vi "Read Multi Eval Meas ES Flatness Results.vi"(8 "error in (no error)":errorcluster, 9 "Result Type (Current)":i32(ring) items=["Current", "Average", "Extreme", "Standard Deviation"], 10 "Instance (1)":T2=1, 11 "VISA resource name":refnum<visa-resource-name>) -> (0 "error out":errorcluster, 1 "Flatness Results":T1 {"Max R2" format="%^.3e"; "Min R2" format="%^.3e"; "Max R1" format="%^.3e"; "Min R1" format="%^.3e"; "Max R2 Min R1" format="%^.3e"; "Max R1 Min R2" format="%^.3e"; "Ripple 2" format="%^.3e"; "Ripple 1" format="%^.3e"}, 2 "Reliability":i32, 3 "VISA resource name out":refnum<visa-resource-name>, 5 "Out Of Tolerance":i32)   [LabVIEW 2020, in "Rohde&Schwarz CMWXP NR FR1 Measurement.lvlib"]
doc: "Return current, average, extreme and standard deviation single value results of the equalizer spectrum flatness measurement.\n\nAttributes:\nRSCMWXPNRFR1M_ATTR_READ_MULTI_EVAL_MEAS_ES_FLATNESS_CURRENT_RESULTS\nRSCMWXPNRFR1M_ATTR_READ_MULTI_EVAL_MEAS_ES_FLATNESS_AVERAGE_RESULTS\nRSCMWXPNRFR1M_ATTR_READ_MULTI_EVAL_MEAS_ES_FLATNESS_EXTREME_RESULTS\nRSCMWXPNRFR1M_ATTR_READ_MULTI_EVAL_MEAS_ES_FLATNESS_STANDARD_DEVIATION_RESULTS\n\nRemote-control commands:\nREAD:NRSub:MEAS<i>:MEValuation:ESFLatness:CURRent?\nREAD:NRSub:MEAS<i>:MEValuation:ESFLatness:AVERage?\nREAD:NRSub:MEAS<i>:MEValuation:ESFLatness:EXTReme?\nREAD:NRSub:MEAS<i>:MEValuation:ESFLatness:SDEViation?"
uses:
  <instrlib>/Rohde&Schwarz CMWXP NR FR1 Measurement/Rohde&Schwarz CMWXP NR FR1 Measurement.lvlib
  <instrlib>/Rohde&Schwarz CMWXP NR FR1 Measurement/Private/_Instance.ctl
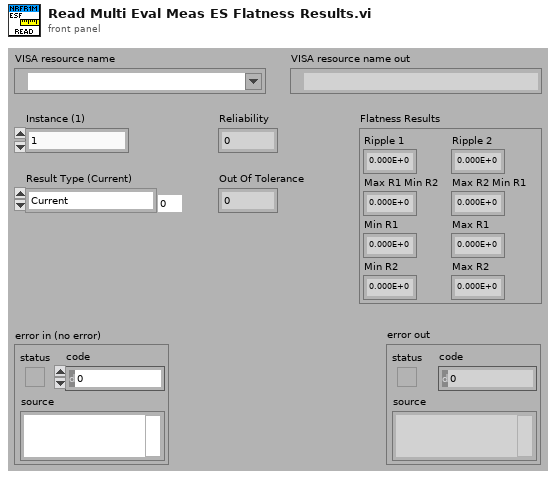
[diagram p1: front panel]
types:
  T1 = cluster{"Ripple 1":dbl, "Ripple 2":dbl, "Max R1 Min R2":dbl, "Max R2 Min R1":dbl, "Min R1":dbl, "Max R1":dbl, "Min R2":dbl, "Max R2":dbl}
  T2 = typedef "Rohde&Schwarz CMWXP NR FR1 Measurement.lvlib/_Instance.ctl" = i32
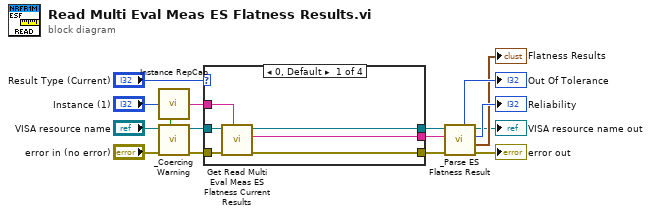
[diagram p0: block diagram]
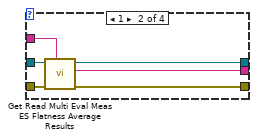
[diagram p2: hidden frame]
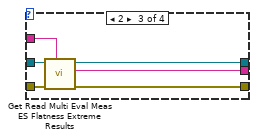
[diagram p3: hidden frame]
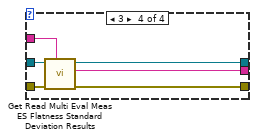
[diagram p4: hidden frame]
diagram:
  n1 = call <instrlib>:"Instance RepCap.vi"("Instance In"="Instance (1)") -> ("In Range?"=w14:bool, "RepCap Identifier Out"=w12:string)  [unwired: 1 in]
  n2 = call <instrlib>:"_Coercing Warning.vi"("In Range?"=w14, "error in (no error)"="error in (no error)", "VISA resource name"="VISA resource name") -> ("error out"=w10:errorcluster, "VISA resource name out"=w11:refnum<visa-resource-name>)  [unwired: 7 in]
  n3 = case shown="0, Default" "Result Type (Current)" {
    tunnel: w12 -> [w22 w28 w34 w40]
    tunnel: w11 -> [w21 w27 w33 w39]
    tunnel: w10 -> [w20 w26 w32 w38]
    tunnel: [w19 w25 w31 w37] -> w6
    tunnel: [w18 w24 w30 w36] -> w7
    tunnel: [w17 w23 w29 w35] -> w8
    frame 0, Default {
      n4 = call "Get Read Multi Eval Meas ES Flatness Current Results"("Repeated Capabilities"=w22, "error in (no error)"=w20, "instrument handle"=w21) -> ("error out"=w17:errorcluster, "Read Multi Eval Meas ES Flatness Current Results"=w18:string, "instrument handle out"=w19:refnum<visa-resource-name>)  [unwired: 6 in]
    }
    frame 1 {
      n5 = call "Get Read Multi Eval Meas ES Flatness Average Results"("Repeated Capabilities"=w28, "error in (no error)"=w26, "instrument handle"=w27) -> ("error out"=w23:errorcluster, "Read Multi Eval Meas ES Flatness Average Results"=w24:string, "instrument handle out"=w25:refnum<visa-resource-name>)  [unwired: 6 in]
    }
    frame 2 {
      n6 = call "Get Read Multi Eval Meas ES Flatness Extreme Results"("Repeated Capabilities"=w34, "error in (no error)"=w32, "instrument handle"=w33) -> ("error out"=w29:errorcluster, "Read Multi Eval Meas ES Flatness Extreme Results"=w30:string, "instrument handle out"=w31:refnum<visa-resource-name>)  [unwired: 6 in]
    }
    frame 3 {
      n7 = call "Get Read Multi Eval Meas ES Flatness Standard Deviation Results"("Repeated Capabilities"=w40, "error in (no error)"=w38, "instrument handle"=w39) -> ("error out"=w35:errorcluster, "Read Multi Eval Meas ES Flatness Standard Deviation Results"=w36:string, "instrument handle out"=w37:refnum<visa-resource-name>)  [unwired: 6 in]
    }
  }
  n8 = call <instrlib>:"_Parse ES Flatness Result.vi"("error in (no error)"=w8, "Input String"=w7, "VISA resource name"=w6) -> ("error out"=→"error out":errorcluster, "Flatness Results"=→"Flatness Results":T1, "Reliability"=→"Reliability":i32, "VISA resource name out"=→"VISA resource name out":refnum<visa-resource-name>, "Out Of Tolerance"=→"Out Of Tolerance":i32)  [unwired: 4 in]
